vi "ResizeColumns.vi"(8 "error in (no error)":errorcluster, 11 "AdjustableMulticolumnListbox in":refnum<class "AdjMCLB.lvclass">) -> (0 "error out":errorcluster, 3 "AdjustableMulticolumnListbox out":refnum<class "AdjMCLB.lvclass">)   [LabVIEW 2020, in "AdjMCLB.lvclass"]
uses:
  AdjMCLB.lvclass
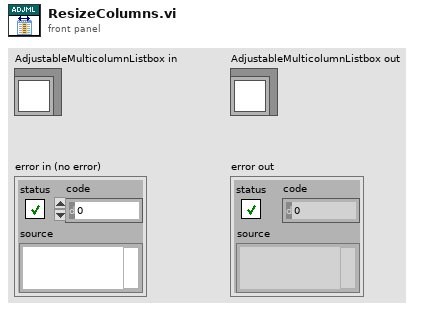
[diagram p1: front panel]
types:
  T1 = typedef "LVBoundsTypeDef.ctl" = cluster{"Width":u32, "Height":u32}
  T2 = typedef "LVRowAndColumnTypeDef.ctl" = cluster{"Row":i32, "Column":i32}
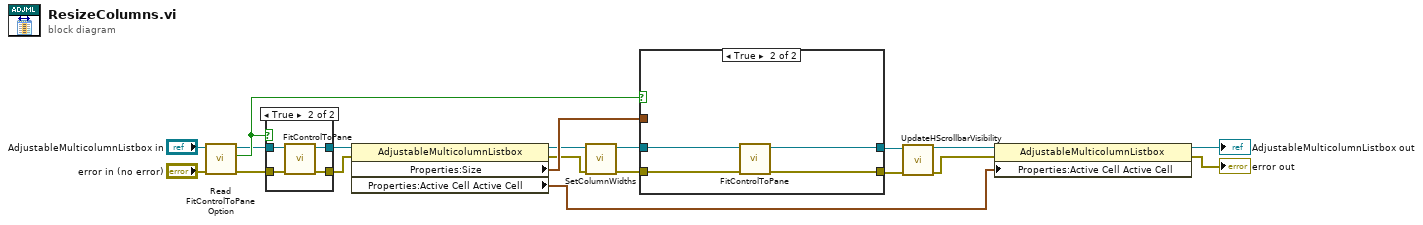
[diagram p0: block diagram]
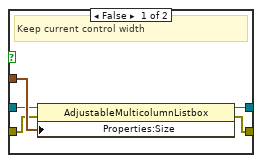
[diagram p3: hidden frame]
diagram:
  n1 = call-dynamic "Read FitControlToPane Option.vi"("error in (no error)"="error in (no error)", "AdjustableMulticolumnListbox in"="AdjustableMulticolumnListbox in") -> ("error out"=w14:errorcluster, "FitControlToPane Option"=w18:bool, "AdjustableMulticolumnListbox out"=w13:refnum<class "AdjMCLB.lvclass">)  [unwired: 7 in]
  n2 = case shown="True" w18 {
    tunnel: w13 -> [w21 w25]
    tunnel: [w21 w24] -> w16
    tunnel: [w20 w23] -> w15
    tunnel: w14 -> [w20 w22]
    frame False {
    }
    frame True {
      n3 = call-dynamic "FitControlToPane.vi"("error in (no error)"=w22, "Control in"=w25) -> ("error out"=w23:errorcluster, "Control out"=w24:refnum<class "AdjMCLB.lvclass">)  [unwired: 8 in]
    }
  }
  n4 = property class="AdjustableMulticolumnListbox"(reference=w16, error in=w15) -> (reference out=w10:refnum<class "AdjMCLB.lvclass">, error out=w9:errorcluster, "Properties:Size"=w19:T1, "Properties:Active Cell Active Cell"=w12:T2)
  n5 = call "SetColumnWidths.vi"("error in (no error)"=w9, "AdjustableMulticolumnListbox in"=w10) -> ("error out"=w5:errorcluster, "AdjustableMulticolumnListbox out"=w6:refnum<class "AdjMCLB.lvclass">)  [unwired: 8 in]
  n6 = case shown="True" w18 {
    tunnel: [w30 w34] -> w4
    tunnel: w19 -> [w29 _]
    tunnel: w6 -> [w28 w33]
    tunnel: w5 -> [w27 w32]
    tunnel: [w26 w31] -> w3
    frame False {
      # "Keep current control width"
      n7 = property class="AdjustableMulticolumnListbox"(reference=w28, error in=w27, "Properties:Size"=w29) -> (reference out=w30:refnum<class "AdjMCLB.lvclass">, error out=w26:errorcluster)
    }
    frame True {
      n8 = call-dynamic "FitControlToPane.vi"("error in (no error)"=w32, "Control in"=w33) -> ("error out"=w31:errorcluster, "Control out"=w34:refnum<class "AdjMCLB.lvclass">)  [unwired: 8 in]
    }
  }
  n9 = call "UpdateHScrollbarVisibility.vi"("error in (no error)"=w3, "AdjustableMulticolumnListbox in"=w4) -> ("error out"=w2:errorcluster, "AdjustableMulticolumnListbox out"=w1:refnum<class "AdjMCLB.lvclass">)  [unwired: 8 in]
  n10 = property class="AdjustableMulticolumnListbox"(reference=w1, error in=w2, "Properties:Active Cell Active Cell"=w12) -> (reference out=→"AdjustableMulticolumnListbox out":refnum<class "AdjMCLB.lvclass">, error out=→"error out":errorcluster)
